vi "ReadTxBuffer.vi"(8 "error in":errorcluster, 11 "Python":T1) -> (0 "error out":errorcluster, 1 "Tx Buffer":string, 2 "Tx Buffer Len":string, 3 "Python":T1)   [LabVIEW 2022 SP3]
uses:
  PythonCtrl.ctl
  Processors.ctl
panel:
  out "tx_len":u32
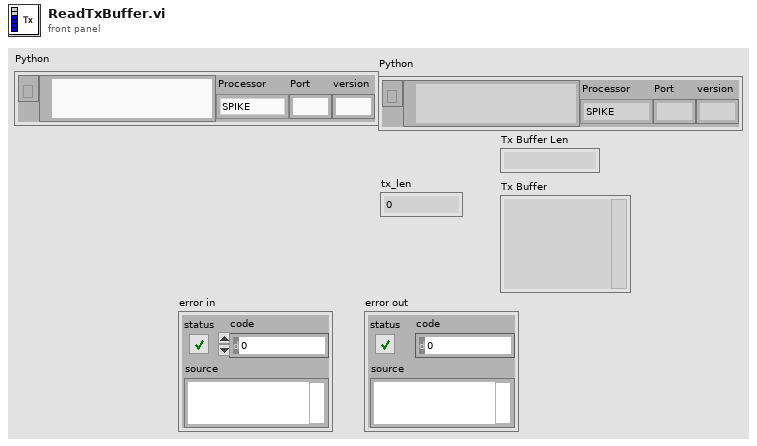
[diagram p1: front panel]
types:
  T1 = typedef "PythonCtrl.ctl" = cluster{"session":refnum<k35>, "PyPath":path, "Processor":T2, "Port":string, "version":string}
  T2 = typedef "Processors.ctl" = enum16{"SPIKE", "Pi", "Pi_ssh", "OpenMV", "Dunio"}
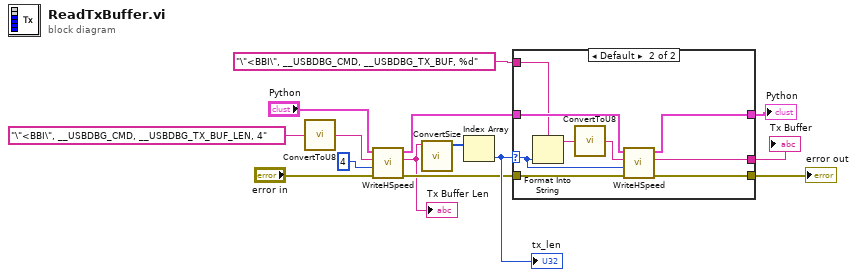
[diagram p0: block diagram]
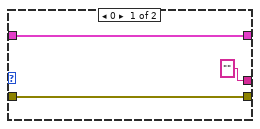
[diagram p2: hidden frame]
diagram:
  n1 = call "ConvertToU8.vi"("struct"="\"<BBI\", __USBDBG_CMD, __USBDBG_TX_BUF_LEN, 4" ("write buffer")) -> ("Binary"=w12:string)
  n2 = call "WriteHSpeed.vi"("error in"="error in", "Reply length"=4, "write buffer"=w12, "Python"="Python") -> ("error out"=w8:errorcluster, "read buffer"=w4:string, "Python"=w6:T1)  [unwired: 5 in]
  "Tx Buffer Len" <- w4
  n3 = call "ConvertSize.vi"("read buffer"=w4) -> ("size()"=w5:u32[])  [unwired: 9 in, 1 out]
  n4 = Index Array(array=w5) -> (element=w14:u32)  [unwired: 1 in]
  "tx_len" <- w14
  n5 = case shown="Default" w14 {
    selector: w14 -> [_ w19]
    tunnel: w6 -> [w17 w26]
    tunnel: w8 -> [w16 w25]
    tunnel: [w16 w24] -> w9
    tunnel: [w17 w23] -> w10
    tunnel: "\"<BBI\", __USBDBG_CMD, __USBDBG_TX_BUF, %d" ("write buffer") -> [_ w22]
    tunnel: ["" ("read buffer") w18] -> w1
    frame 0 {
    }
    frame Default {
      n6 = Format Into String(format string=w22, w19) -> (resulting string=w21:string)  [unwired: 2 in, 1 out]
      n7 = call "ConvertToU8.vi"("struct"=w21) -> ("Binary"=w20:string)
      n8 = call "WriteHSpeed.vi"("error in"=w25, "Reply length"=w19, "write buffer"=w20, "Python"=w26) -> ("error out"=w24:errorcluster, "read buffer"=w18:string, "Python"=w23:T1)  [unwired: 5 in]
    }
  }
  "Tx Buffer" <- w1
  "Python" <- w10
  "error out" <- w9
